vi "Relative Standard Deviation.vi"(11 "Input Array":dbl[](array[numeric])) -> (1 "Relative Standard Deviation":dbl, 3 "Relative Standard Deviation":string)   [LabVIEW 2014]
uses:
  <vilib>/Analysis/NI_AALBase.lvlib
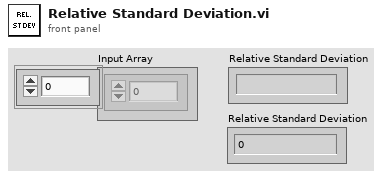
[diagram p1: front panel]
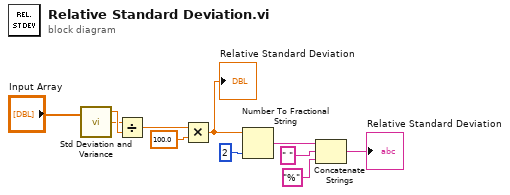
[diagram p0: block diagram]
diagram:
  n1 = call <vilib>:"Std Deviation and Variance.vi"("X"="Input Array") -> ("mean"=w3:dbl, "standard deviation"=w2:dbl)  [unwired: 1 in, 1 out]
  n2 = Divide(x=w2, y=w3) -> (x/y=w4:dbl)
  n3 = Multiply(x=w4, y=100.0) -> (x*y=w6:dbl)
  "Relative Standard Deviation" <- w6
  n4 = Number To Fractional String(number=w6, precision (6)=i16 2) -> (F-format string=w8:string)  [unwired: 2 in]
  n5 = Concatenate Strings(w8, " " ("string"), "%" ("string")) -> (→"Relative Standard Deviation":string)
